vi "Stop.vi"() -> ()   [LabVIEW 2015]
panel:
  out "stop":bool
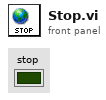
[diagram p1: front panel]
diagram:
